vi "按日保存每天数据.vi"(2 "列首":string[](array[string])=["序号", "时间", "作业员编号", "设备编号", "电池条码1", "查询结果1", "电池条码2", "查询结果2"], 4 "保存内容":string[](array[string])=["序号", "时间", "作业员编号", "设备编号", "电池条码1", "查询结果1", "电池条码2", "查询结果2"], 5 "保存路径":path=path "d:/弹夹管控上传数据") -> (0 "error out 3":errorcluster, 1 "每天保存路径":path)   [LabVIEW 2020]
uses:
  <vilib>/Utility/file.llb/Write To Spreadsheet File (string).vi
panel:
  out "error out 2":errorcluster caption="错误输出"
  out "错误输出 2":errorcluster caption="错误输出"
  out "错误输出":errorcluster
  out "error out":errorcluster caption="错误输出"
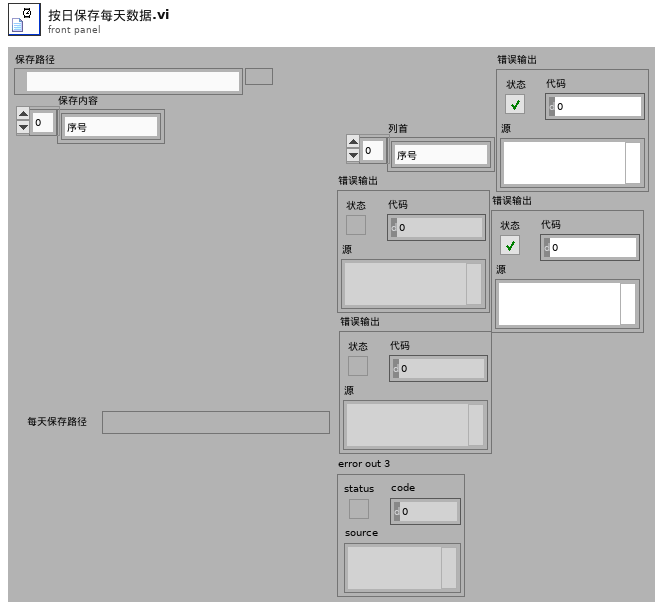
[diagram p1: front panel]
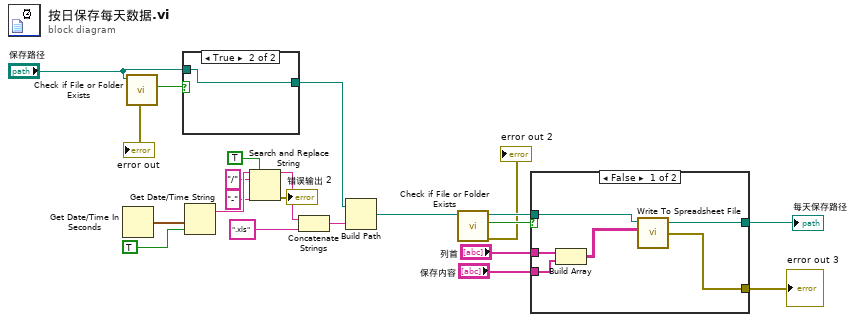
[diagram p0: block diagram]
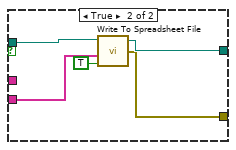
[diagram p2: hidden frame]
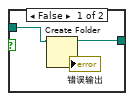
[diagram p3: hidden frame]
diagram:
  n1 = Get Date/Time In Seconds() -> (seconds since 1Jan1904=w18:timestamp)
  n2 = call <vilib>:"Check if File or Folder Exists.vi"("path"="保存路径") -> ("error out"=→"error out":errorcluster, "file or folder exists?"=w22:bool)  [unwired: 8 in, 1 out]
  n3 = case shown="True" w22 {
    tunnel: "保存路径" -> [w25 w26]
    tunnel: [w24 w26] -> w11
    frame False {
      n4 = Create Folder(path (use dialog)=w25) -> (created path=w24:path, error out=→"错误输出":errorcluster)  [unwired: 2 in, 1 out]
    }
    frame True {
    }
  }
  n5 = Get Date/Time String(seconds (now)=w18, want seconds? (F)=TRUE ("需要秒？(F)")) -> (date string=w16:string)  [unwired: 1 in, 1 out]
  n6 = Search and Replace String(replace all?=TRUE ("替换全部？(F)"), input string=w16, search string="/" ("搜索字符串"), replace string="-" ("替换字符串(\"\")")) -> (result string=w12:string, error out=→"错误输出 2":errorcluster)  [unwired: 4 in, 2 out]
  n7 = Concatenate Strings(w12, ".xls" ("字符串")) -> (w21:string)
  n8 = Build Path(base path=w11, name or relative path=w21) -> (appended path=w10:path)
  n9 = call <vilib>:"Check if File or Folder Exists.vi"("path"=w10) -> ("error out"=→"error out 2":errorcluster, "file or folder exists?"=w9:bool, "dup path"=w8:path)  [unwired: 8 in]
  n10 = case shown="False" w9 {
    tunnel: w8 -> [w29 w37]
    tunnel: "保存内容" -> [w31 w36]
    tunnel: "列首" -> [w32 _]
    tunnel: [w28 w34] -> w5
    tunnel: [w27 w33] -> w1
    frame False {
      n11 = Build Array(w32, w31) -> (w30:string[][])
      n12 = call-poly <vilib>:"Write To Spreadsheet File.vi"("2D data"=w30, "file path (dialog if empty)"=w29) -> ("error out"=w27:errorcluster, "new file path (Not A Path if cancelled)"=w28:path)  [unwired: 5 in]
    }
    frame True {
      n13 = call-poly <vilib>:"Write To Spreadsheet File.vi"("append to file? (new file:F)"=TRUE, "1D data"=w36, "file path (dialog if empty)"=w37) -> ("error out"=w33:errorcluster, "new file path (Not A Path if cancelled)"=w34:path)  [unwired: 4 in]
    }
  }
  "每天保存路径" <- w5
  "error out 3" <- w1
